vi "Create-S-Box-Number.vi"(11 "Index":u8=3 format="%x") -> (3 "S-Box":u8 format="%x")   [LabVIEW 2017]
panel:
  out "Inverse":u8 format="%x"
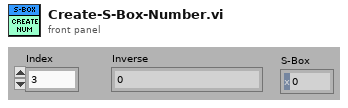
[diagram p1: front panel]
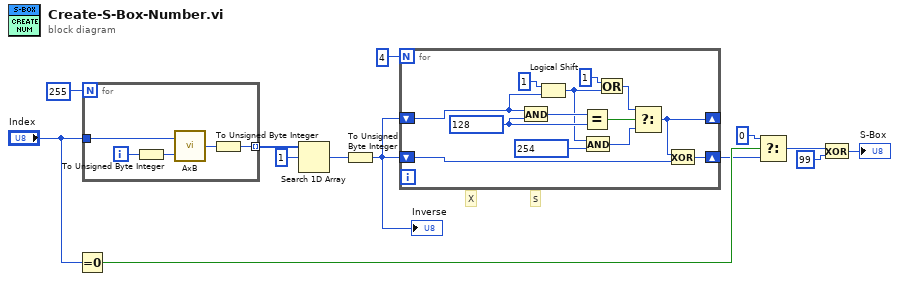
[diagram p0: block diagram]
diagram:
  # "X"
  # "S"
  n1 = Equal To 0?(x="Index") -> (x = 0?=w3:bool)
  n2 = for {
    N: 255 -> [_]
    tunnel: "Index" -> [w17]
    tunnel: [w15] -> w10 mode=indexing
    i -> [w18]
    n3 = To Unsigned Byte Integer(number=w18) -> (unsigned 8bit integer=w14:u8)
    n4 = call "AxB.vi"("B"=w14, "A"=w17) -> ("Numeric"=w16:u8)
    n5 = To Unsigned Byte Integer(number=w16) -> (unsigned 8bit integer=w15:u8)
  }
  n6 = Search 1D Array(1D array=w10, element=u8 1) -> (index of element=w8:i32)  [unwired: 1 in]
  n7 = To Unsigned Byte Integer(number=w8) -> (unsigned 8bit integer=w7:u8)
  "Inverse" <- w7
  n8 = for {
    N: 4 -> [_]
    shift-right: [w21] -> _
    shift-left: w7 -> [w29]
    shift-right: [w19] -> w2
    shift-left: w7 -> [w20]
    w30 = u8 128 ("y")
    n9 = And(x=w29, y=w30) -> (x .and. y?=w31:u8)
    n10 = Logical Shift(y=u8 1, x=w29) -> (x << y=w26:u8)
    n11 = Equal?(x=w31, y=w30) -> (x = y?=w23:bool)
    n12 = And(x=w26, y=u8 254) -> (x .and. y?=w24:u8)
    n13 = Or(x=u8 1 ("y"), y=w26) -> (x .or. y?=w22:u8)
    n14 = Select(t=w22, s=w23, f=w24) -> (s? t:f=w21:u8)
    n15 = Exclusive Or(1:w20, 2:w21) -> (0:w19:u8)
  }
  n16 = Select(t=u8 0, s=w3, f=w2) -> (s? t:f=w5:u8)
  n17 = Exclusive Or(1:u8 99 ("y"), 2:w5) -> (0:→"S-Box":u8)
